vi "Update Selected Channels.vi"(8 "error in":errorcluster, 9 "Channel Refs":T1[](array[typedef]) format="%.0x", 10 "Channel Names":string[](array[string]), 11 "Listbox":refnum<vi>) -> (0 "error out":errorcluster)   [LabVIEW 2024, in "Nominal Client System Explorer.lvlib"]
uses:
  <vilib>/NI VeriStand/Custom Device API/Custom Device Item Ref.ctl
  <vilib>/Utility/miscctls.llb/LVRowAndColumnUnsignedTypeDef.ctl
  Nominal Client System Explorer.lvlib
  <vilib>/NI VeriStand/Custom Device API/Custom Device API.lvlib
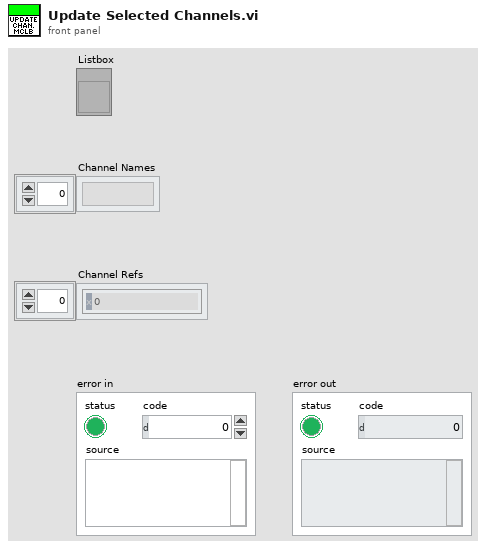
[diagram p1: front panel]
types:
  T1 = typedef "Custom Device API.lvlib/Custom Device Item Ref.ctl" = u64
  T2 = typedef "LVRowAndColumnUnsignedTypeDef.ctl" = cluster{"Row":u32, "Column":u32}
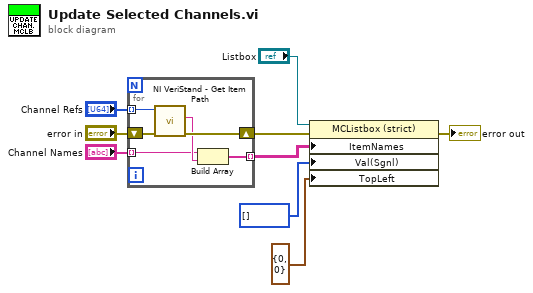
[diagram p0: block diagram]
diagram:
  n1 = for {
    shift-right: [w13] -> w6
    shift-left: "error in" -> [w15]
    tunnel: "Channel Refs" -> [w14] mode=indexing
    tunnel: [w11] -> w7 mode=indexing
    tunnel: "Channel Names" -> [w10] mode=indexing
    n2 = call <vilib>:"NI VeriStand - Get Item Path.vi"("error in (no error)"=w15, "Item Ref in"=w14) -> ("error out"=w13:errorcluster, "Path"=w12:string)  [unwired: 8 out]
    n3 = Build Array(w10, w12) -> (w11:string[])
  }
  n4 = property on="Property Node" class="MCListbox (strict)"(reference="Listbox", error in=w6, "ItemNames"=w7, "Val(Sgnl)"=i32[] [] ("Value (Signaling)"), "TopLeft"=T2 {"Row"=0, "Column"=0} ("Top Left Visible Cell")) -> (error out=→"error out":errorcluster)  [unwired: 1 out]
